vi "Teleop.vi"(10 "Match Info":T1={"Autonomous Elapsed Seconds"=0.0, "TeleOp Elapsed Seconds"=0.0, "Disabled Elapsed Seconds"=0.0, "Visited Autonomous"=FALSE, "Visited TeleOp"=FALSE, "Visited Disabled"=FALSE, "Autonomous Settings"={"Autonomous Style"=enum."Independent", "VI Refnum"=refnum}}, 11 "Call Context":T2) -> ()   [LabVIEW 2012]
doc: "This VI is called for each TeleOp packet received from the DS where the robot is not disabled. It is often used to read from the joysticks and update I/O or to update setpoints for timed control loops. It should complete and return within 20 milliseconds or it may miss DS packets."
uses:
  <vilib>/Rock Robotics/WPI/DriverStation/WPI_DriverStationDerivedRobotMode.ctl
  <vilib>/Rock Robotics/WPI/DriverStation/WPI_DriverStationMatch Info.ctl
  <vilib>/Rock Robotics/WPI/Solenoid/WPI_SolenoidValue.ctl
  Robot Global Data.vi
  <vilib>/Rock Robotics/WPI/Solenoid/WPI_SolenoidSetEnum.vi
  <vilib>/Rock Robotics/WPI/Joystick/WPI_JoystickGetSetRefNum.vi
  <vilib>/Rock Robotics/WPI/RobotDrive/WPI_RobotDriveGetSetRefNum.vi
panel:
  in  "Spin 2":dbl=0.75
  in  "Shoot 2":dbl=1.0
  in  "Spin":dbl=0.75
  in  "Shoot":dbl=1.0
  out "Numeric 1":dbl(slide) scale=0.0..100.0
  out "Boolean 2":bool
  out "Boolean 1":bool
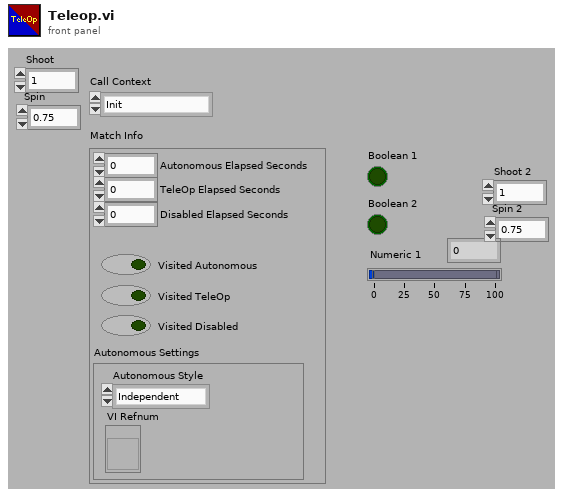
[diagram p1: front panel]
types:
  T1 = typedef "WPI_DriverStationMatch Info.ctl" = cluster{"Autonomous Elapsed Seconds":dbl, "TeleOp Elapsed Seconds":dbl, "Disabled Elapsed Seconds":dbl, "Visited Autonomous":bool, "Visited TeleOp":bool, "Visited Disabled":bool, "Autonomous Settings":cluster{"Autonomous Style":enum16{"Iterative", "Independent"}, "VI Refnum":refnum<vi>}}
  T2 = typedef "WPI_DriverStationDerivedRobotMode.ctl" = enum16{"Init", "Execute", "Stop"}
  T3 = typedef "WPI_SolenoidValue.ctl" = enum16{"Off", "On", "Forward", "Reverse"}
  T4 = typedef "WPI_RobotDriveDevRef.ctl" = cluster{"DevStatus":errorcluster, "Motors[]":T5[], "Square Inputs":bool, "Max Output":dbl, "Isochronous":bool}
  T5 = typedef "WPI_MotorControlDeviceRef.ctl" = cluster{"DeviceStatus":errorcluster, "Type":enum16{"PWM", "CAN"}, "PWM":cluster{"Digital Module":T6, "PWM Channel":T7, "DeadBand":T8}, "CAN":cluster{"Device Number":u8, "Control Mode":T9, "Semaphore":T10, "Max Vout":dbl}, "Invert":bool, "TransformRef":T11, "InvTransformRef":T11}
  T6 = typedef "FPGA_TypedefDigitalModule.ctl" = enum16{"Digital Module 1", "Digital Module 2"}
  T7 = typedef "FPGA_DIOPWMChannel.ctl" = enum8{"PWM 1", "PWM 2", "PWM 3", "PWM 4", "PWM 5", "PWM 6", "PWM 7", "PWM 8", "PWM 9", "PWM 10", "Invalid"}
  T8 = typedef "WPI_PWMDeadband.ctl" = cluster{"Name":string, "maxPositivePwm":i32, "minPositivePwm":i32, "centerPwm":i32, "maxNegativePwm":i32, "minNegativePwm":i32, "angularRange":u16}
  T9 = typedef "WPI_CANJaguar_ControlMode.ctl" = enum8{"Percent VBus", "Current", "Speed", "Position", "Voltage"}
  T10 = typedef "Semaphore RefNum" = refnum<k1>
  T11 = typedef "WPI_PWMTransform_ConPane.ctl" = refnum<vi>
  T12 = typedef "WPI_JoystickDevRef.ctl" = cluster{"Device":T13}
  T13 = typedef "WPI_JoystickDeviceEnum.ctl" = enum16{"USB 1", "USB 2", "USB 3", "USB 4", "Kinect 1", "Kinect 2"}
  T14 = typedef "WPI_JoystickButtonState.ctl" = cluster{"Button 1":bool, "Button 2":bool, "Button 3":bool, "Button 4":bool, "Button 5":bool, "Button 6":bool, "Button 7":bool, "Button 8":bool, "Button 9":bool, "Button 10":bool, "Button 11":bool, "Button 12":bool}
  T15 = cluster{"axis 1 (x)":dbl, "axis 2 (y)":dbl, "axis 3 (throttle)":dbl, "axis 4":dbl, "axis 5":dbl, "axis 6":dbl}
  T16 = typedef "WPI_SolenoidDevRef.ctl" = cluster{"DevStatus":errorcluster, "Solenoid Module":T17, "Forward Solenoid Channel":T18, "Reverse Solenoid Channel":T18}
  T17 = typedef "FPGA_TypedefSolenoidModule.ctl" = enum16{"Solenoid Module 1", "Solenoid Module 2"}
  T18 = typedef "WPI_SolenoidChannel.ctl" = enum8{"Solenoid 1", "Solenoid 2", "Solenoid 3", "Solenoid 4", "Solenoid 5", "Solenoid 6", "Solenoid 7", "Solenoid 8", "Invalid"}
  T19 = typedef "WPI_GyroDevRef.ctl" = cluster{"DevStatus":errorcluster, "Analog Module":T20, "Analog Channel":T21, "Offset":dbl, "Gain (VoltsPerDegree/Second)":dbl}
  T20 = typedef "FPGA_TypedefAnalogModule.ctl" = enum16{"Analog Module 1", "Analog Module 2"}
  T21 = typedef "FPGA_AIChannel.ctl" = enum8{"AI 1", "AI 2", "AI 3", "AI 4", "AI 5", "AI 6", "AI 7", "AI 8", "Invalid"}
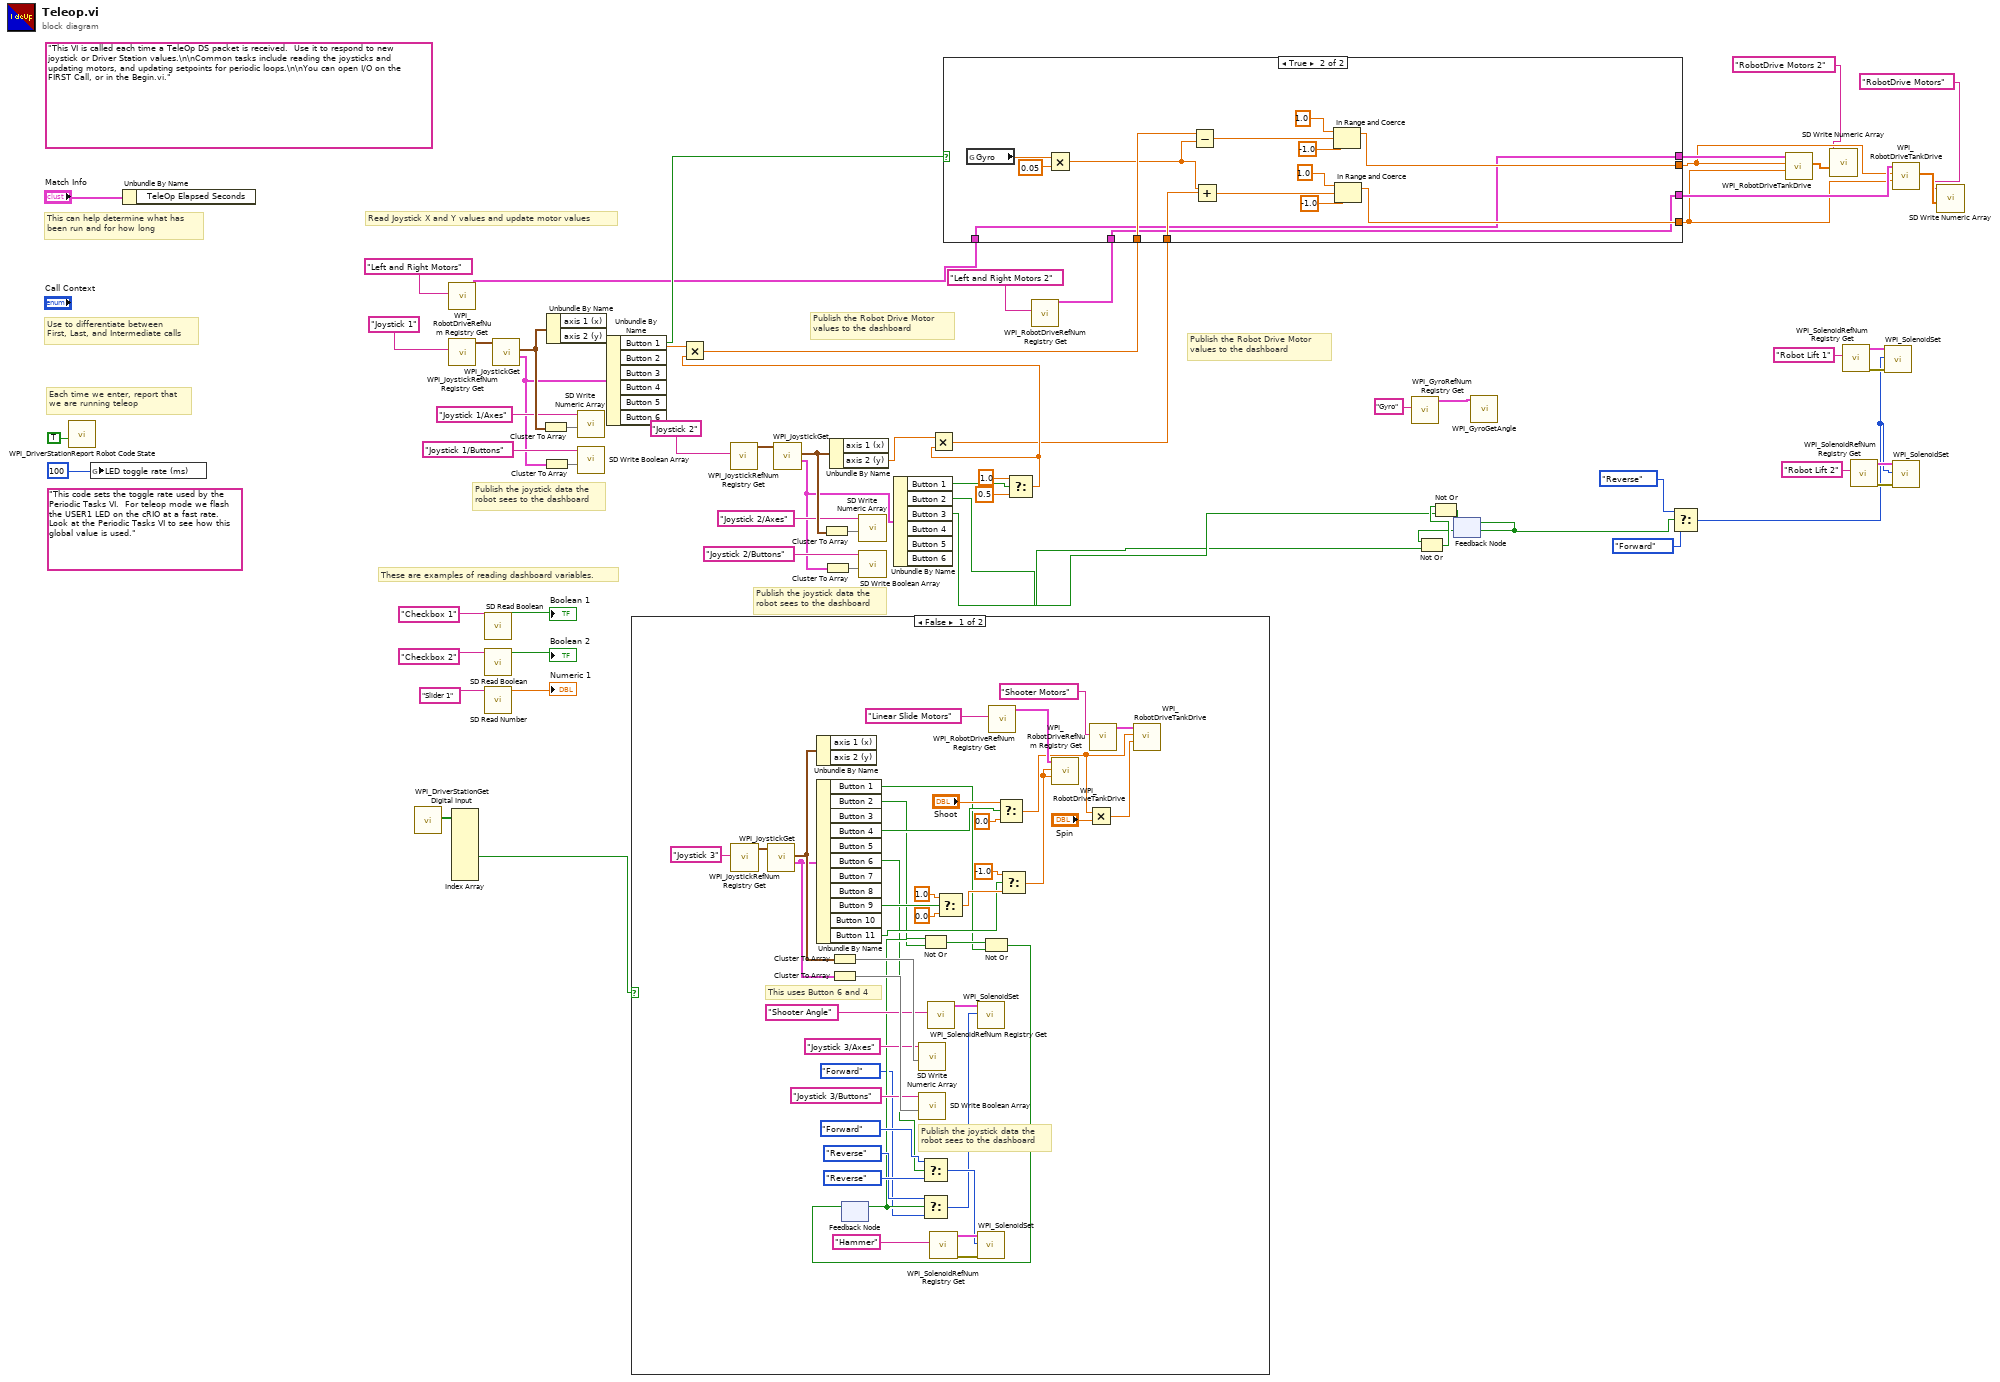
[diagram p0: block diagram]
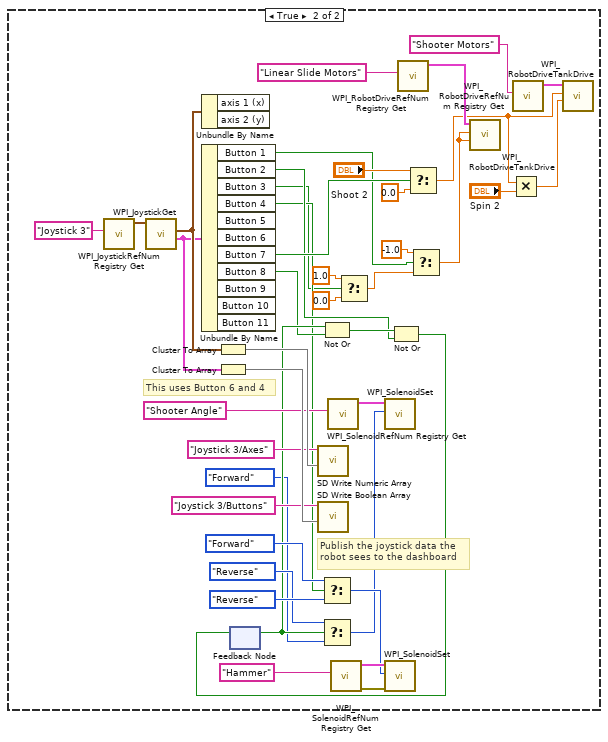
[diagram p2: hidden frame]
diagram:
  (unwired) "This code sets the toggle rate used by the Periodic Tasks VI.  For teleop mode we flash the USER1 LED on the cRIO at a fast rate.  Look at the Periodic Tasks VI to see how this global value is used."
  (unwired) "This VI is called each time a TeleOp DS packet is received.  Use it to respond to new joystick or Driver Station values.\n\nCommon tasks include reading the joysticks and updating motors, and updating setpoints for periodic loops.\n\nYou can open I/O on the FIRST Call, or in the Begin.vi."
  # "Publish the Robot Drive Motor\nvalues to the dashboard"
  # "Publish the joystick data the\nrobot sees to the dashboard"
  # "These are examples of reading dashboard variables."
  # "Publish the Robot Drive Motor\nvalues to the dashboard"
  # "Publish the joystick data the\nrobot sees to the dashboard"
  # "Each time we enter, report that\nwe are running teleop"
  # "Use to differentiate between\nFirst, Last, and Intermediate calls"
  # "This can help determine what has\nbeen run and for how long"
  # "Read Joystick X and Y values and update motor values"
  n1 = call <vilib>:"WPI_DriverStationReport Robot Code State.vi"("TeleOp"=TRUE ("Autonomous")) -> ()  [unwired: 10 in, 1 out]
  n2 = global write "Robot Global Data.vi" "LED toggle rate (ms)"(u32 100 ("LED ms toggle rate")) -> ()
  n3 = Unbundle By Name("Match Info") -> ()  [unwired: 1 out]
  n4 = call <vilib>:"WPI_DriverStationGet Digital Input.vi"() -> ("Driver Station Digital Input (1-8)"=w2:bool[])  [unwired: 11 out]
  n5 = call <vilib>:"WPI_RobotDriveRefNum Registry Get.vi"("refnum name"="Left and Right Motors") -> ("RobotDriveDevRef"=w17:T4)  [unwired: 1 in, 9 out]
  n6 = call <vilib>:"WPI_JoystickRefNum Registry Get.vi"("refnum name"="Joystick 1") -> ("JoystickDevRef"=w61:T12)  [unwired: 1 in, 9 out]
  n7 = Index Array(array=w2) -> (element #5=w1:bool)  [unwired: 8 in, 7 out]
  n8 = call <vilib>:"SD Read Boolean.vi"("Name"="Checkbox 1" ("refnum name")) -> ("Boolean"=→"Boolean 1":bool)  [unwired: 8 in, 2 out]
  n9 = call <vilib>:"SD Read Boolean.vi"("Name"="Checkbox 2" ("refnum name")) -> ("Boolean"=→"Boolean 2":bool)  [unwired: 8 in, 2 out]
  n10 = call <vilib>:"SD Read Number.vi"("Name"="Slider 1" ("refnum name")) -> ("Numeric"=→"Numeric 1":dbl)  [unwired: 8 in, 2 out]
  n11 = call <vilib>:"WPI_JoystickGet.vi"("JoystickDevRef"=w61) -> ("Buttons"=w19:T14, "Axes"=w56:T15)  [unwired: 1 in, 4 out]
  n12 = Cluster To Array(cluster=w56) -> (array=w55:dbl[])
  n13 = Cluster To Array(cluster=w19) -> (array=w58:bool[])
  n14 = Unbundle By Name(w56) -> ("axis 2 (y)"=w35:dbl)  [unwired: 1 out]
  n15 = call <vilib>:"SD Write Numeric Array.vi"("Numeric Array"=w55, "Name"="Joystick 1/Axes") -> ()  [unwired: 8 in, 2 out]
  n16 = call <vilib>:"SD Write Boolean Array.vi"("Boolean Array"=w58, "Name"="Joystick 1/Buttons") -> ()  [unwired: 8 in, 2 out]
  n17 = Unbundle By Name(w19) -> ("Button 1"=w18:bool)  [unwired: 5 out]
  n18 = case shown="False" w1 {
    frame False {
      # "This uses Button 6 and 4"
      # "Publish the joystick data the\nrobot sees to the dashboard"
      n19 = call <vilib>:"WPI_JoystickRefNum Registry Get.vi"("refnum name"="Joystick 3") -> ("JoystickDevRef"=w104:T12)  [unwired: 1 in, 9 out]
      n20 = call <vilib>:"WPI_JoystickGet.vi"("JoystickDevRef"=w104) -> ("Buttons"=w98:T14, "Axes"=w101:T15)  [unwired: 1 in, 4 out]
      n21 = Unbundle By Name(w101) -> ()  [unwired: 2 out]
      n22 = Unbundle By Name(w98) -> ("Button 1"=w65:bool, "Button 2"=w67:bool, "Button 4"=w68:bool, "Button 6"=w66:bool, "Button 9"=w69:bool, "Button 11"=w93:bool)  [unwired: 5 out]
      n23 = Cluster To Array(cluster=w101) -> (array=w100:dbl[])
      n24 = Cluster To Array(cluster=w98) -> (array=w103:bool[])
      n25 = feedback #1() -> (w71:bool)  [unwired: 1 in]
      n26 = call <vilib>:"SD Write Numeric Array.vi"("Numeric Array"=w100, "Name"="Joystick 3/Axes") -> ()  [unwired: 8 in, 2 out]
      n27 = call <vilib>:"SD Write Boolean Array.vi"("Boolean Array"=w103, "Name"="Joystick 3/Buttons") -> ()  [unwired: 8 in, 2 out]
      n28 = Not Or(1:w67, 2:w71) -> (0:w73:bool)
      n29 = Select(t=WPI_SolenoidValue."Forward" ("Value"), s=w66, f=WPI_SolenoidValue."Reverse" ("Value")) -> (s? t:f=w80:T3)
      n30 = Select(t=WPI_SolenoidValue."Reverse" ("Value"), s=w71, f=WPI_SolenoidValue."Forward" ("Value")) -> (s? t:f=w75:T3)
      n31 = call <vilib>:"WPI_SolenoidRefNum Registry Get.vi"("refnum name"="Shooter Angle") -> ("SolenoidDevRef"=w76:T16)  [unwired: 9 in, 1 out]
      n32 = call <vilib>:"WPI_SolenoidRefNum Registry Get.vi"("refnum name"="Hammer") -> ("error out"=w83:errorcluster, "SolenoidDevRef"=w82:T16)  [unwired: 9 in]
      n33 = Select(t=1.0, s=w69, f=0.0) -> (s? t:f=w94:dbl)
      n34 = call-poly <vilib>:"WPI_SolenoidSet.vi"("Value"=w75, "SolenoidDevRef"=w76) -> ()  [unwired: 8 in, 2 out]
      n35 = call-poly <vilib>:"WPI_SolenoidSet.vi"("error in (no error)"=w83, "Value"=w80, "SolenoidDevRef"=w82) -> ()  [unwired: 7 in, 2 out]
      n36 = Not Or(1:w65, 2:w73) -> (0:w72:bool)
      n37 = feedback-in #1(w72) -> ()
      n38 = call <vilib>:"WPI_RobotDriveRefNum Registry Get.vi"("refnum name"="Linear Slide Motors") -> ("RobotDriveDevRef"=w91:T4)  [unwired: 9 in, 1 out]
      n39 = Select(t="Shoot", s=w68, f=0.0) -> (s? t:f=w85:dbl)
      n40 = Select(t=-1.0, s=w93, f=w94) -> (s? t:f=w92:dbl)
      n41 = call <vilib>:"WPI_RobotDriveTankDrive.vi"("Right axis value"=w92, "Left axis value"=w92, "RobotDriveDevRef"=w91) -> ()  [unwired: 6 in, 3 out]
      n42 = Multiply(x=w85, y="Spin") -> (x*y=w84:dbl)
      n43 = call <vilib>:"WPI_RobotDriveRefNum Registry Get.vi"("refnum name"="Shooter Motors") -> ("RobotDriveDevRef"=w89:T4)  [unwired: 9 in, 1 out]
      n44 = call <vilib>:"WPI_RobotDriveTankDrive.vi"("Right axis value"=w84, "Left axis value"=w85, "RobotDriveDevRef"=w89) -> ()  [unwired: 6 in, 3 out]
    }
    frame True {
      # "This uses Button 6 and 4"
      # "Publish the joystick data the\nrobot sees to the dashboard"
      n45 = call <vilib>:"WPI_JoystickRefNum Registry Get.vi"("refnum name"="Joystick 3") -> ("JoystickDevRef"=w146:T12)  [unwired: 1 in, 9 out]
      n46 = call <vilib>:"WPI_JoystickGet.vi"("JoystickDevRef"=w146) -> ("Buttons"=w140:T14, "Axes"=w143:T15)  [unwired: 1 in, 4 out]
      n47 = Unbundle By Name(w143) -> ()  [unwired: 2 out]
      n48 = Unbundle By Name(w140) -> ("Button 1"=w107:bool, "Button 2"=w110:bool, "Button 3"=w108:bool, "Button 4"=w109:bool, "Button 7"=w112:bool, "Button 8"=w111:bool)  [unwired: 5 out]
      n49 = Cluster To Array(cluster=w143) -> (array=w142:dbl[])
      n50 = Cluster To Array(cluster=w140) -> (array=w145:bool[])
      n51 = feedback #2() -> (w114:bool)  [unwired: 1 in]
      n52 = call <vilib>:"SD Write Numeric Array.vi"("Numeric Array"=w142, "Name"="Joystick 3/Axes") -> ()  [unwired: 8 in, 2 out]
      n53 = call <vilib>:"SD Write Boolean Array.vi"("Boolean Array"=w145, "Name"="Joystick 3/Buttons") -> ()  [unwired: 8 in, 2 out]
      n54 = Not Or(1:w111, 2:w114) -> (0:w116:bool)
      n55 = Select(t=WPI_SolenoidValue."Forward" ("Value"), s=w109, f=WPI_SolenoidValue."Reverse" ("Value")) -> (s? t:f=w123:T3)
      n56 = Select(t=WPI_SolenoidValue."Reverse" ("Value"), s=w114, f=WPI_SolenoidValue."Forward" ("Value")) -> (s? t:f=w118:T3)
      n57 = call <vilib>:"WPI_SolenoidRefNum Registry Get.vi"("refnum name"="Shooter Angle") -> ("SolenoidDevRef"=w119:T16)  [unwired: 9 in, 1 out]
      n58 = call <vilib>:"WPI_SolenoidRefNum Registry Get.vi"("refnum name"="Hammer") -> ("error out"=w126:errorcluster, "SolenoidDevRef"=w125:T16)  [unwired: 9 in]
      n59 = Select(t=1.0, s=w108, f=0.0) -> (s? t:f=w136:dbl)
      n60 = call-poly <vilib>:"WPI_SolenoidSet.vi"("Value"=w118, "SolenoidDevRef"=w119) -> ()  [unwired: 8 in, 2 out]
      n61 = call-poly <vilib>:"WPI_SolenoidSet.vi"("error in (no error)"=w126, "Value"=w123, "SolenoidDevRef"=w125) -> ()  [unwired: 7 in, 2 out]
      n62 = Not Or(1:w110, 2:w116) -> (0:w115:bool)
      n63 = feedback-in #2(w115) -> ()
      n64 = call <vilib>:"WPI_RobotDriveRefNum Registry Get.vi"("refnum name"="Linear Slide Motors") -> ("RobotDriveDevRef"=w134:T4)  [unwired: 9 in, 1 out]
      n65 = Select(t="Shoot 2", s=w112, f=0.0) -> (s? t:f=w128:dbl)
      n66 = Select(t=-1.0, s=w107, f=w136) -> (s? t:f=w135:dbl)
      n67 = call <vilib>:"WPI_RobotDriveTankDrive.vi"("Right axis value"=w135, "Left axis value"=w135, "RobotDriveDevRef"=w134) -> ()  [unwired: 6 in, 3 out]
      n68 = Multiply(x=w128, y="Spin 2") -> (x*y=w127:dbl)
      n69 = call <vilib>:"WPI_RobotDriveRefNum Registry Get.vi"("refnum name"="Shooter Motors") -> ("RobotDriveDevRef"=w132:T4)  [unwired: 9 in, 1 out]
      n70 = call <vilib>:"WPI_RobotDriveTankDrive.vi"("Right axis value"=w127, "Left axis value"=w128, "RobotDriveDevRef"=w132) -> ()  [unwired: 6 in, 3 out]
    }
  }
  n71 = call <vilib>:"WPI_JoystickRefNum Registry Get.vi"("refnum name"="Joystick 2") -> ("JoystickDevRef"=w46:T12)  [unwired: 1 in, 9 out]
  n72 = call <vilib>:"WPI_JoystickGet.vi"("JoystickDevRef"=w46) -> ("Buttons"=w39:T14, "Axes"=w43:T15)  [unwired: 1 in, 4 out]
  n73 = Cluster To Array(cluster=w43) -> (array=w42:dbl[])
  n74 = Cluster To Array(cluster=w39) -> (array=w45:bool[])
  n75 = Unbundle By Name(w43) -> ("axis 2 (y)"=w34:dbl)  [unwired: 1 out]
  n76 = call <vilib>:"SD Write Numeric Array.vi"("Numeric Array"=w42, "Name"="Joystick 2/Axes") -> ()  [unwired: 8 in, 2 out]
  n77 = call <vilib>:"SD Write Boolean Array.vi"("Boolean Array"=w45, "Name"="Joystick 2/Buttons") -> ()  [unwired: 8 in, 2 out]
  n78 = Unbundle By Name(w39) -> ("Button 1"=w38:bool, "Button 2"=w4:bool, "Button 3"=w5:bool)  [unwired: 3 out]
  n79 = Select(t=1.0, s=w38, f=0.5) -> (s? t:f=w33:dbl)
  n80 = Multiply(x=w35, y=w33) -> (x*y=w15:dbl)
  n81 = Multiply(x=w34, y=w33) -> (x*y=w6:dbl)
  n82 = call <vilib>:"WPI_RobotDriveRefNum Registry Get.vi"("refnum name"="Left and Right Motors 2") -> ("RobotDriveDevRef"=w16:T4)  [unwired: 1 in, 9 out]
  n83 = case shown="True" w18 {
    tunnel: w17 -> [w152 w153]
    tunnel: w16 -> [w151 w154]
    tunnel: w15 -> [w150 w162]
    tunnel: [w149 w155] -> w7
    tunnel: [w152 w153] -> w12
    tunnel: [w151 w154] -> w11
    tunnel: [w150 w156] -> w10
    tunnel: w6 -> [w149 w163]
    frame False {
    }
    frame True {
      n84 = global read "Robot Global Data.vi" "Gyro"() -> (w167:dbl)
      n85 = Multiply(x=w167, y=0.05) -> (x*y=w161:dbl)
      n86 = Subtract(x=w162, y=w161) -> (x-y=w160:dbl)
      n87 = Add(x=w161, y=w163) -> (x+y=w157:dbl)
      n88 = In Range and Coerce(upper limit=1.0, x=w160, lower limit=-1.0) -> (coerced(x)=w156:dbl)  [unwired: 1 out]
      n89 = In Range and Coerce(upper limit=1.0, x=w157, lower limit=-1.0) -> (coerced(x)=w155:dbl)  [unwired: 1 out]
    }
  }
  n90 = call <vilib>:"WPI_GyroRefNum Registry Get.vi"("refnum name"="Gyro") -> ("GyroDevRef"=w21:T19)  [unwired: 9 in, 1 out]
  n91 = feedback #3() -> (w22:bool)  [unwired: 1 in]
  n92 = Not Or(1:w4, 2:w22) -> (0:w24:bool)
  n93 = Not Or(1:w5, 2:w24) -> (0:w23:bool)
  n94 = feedback-in #3(w23) -> ()
  n95 = call <vilib>:"WPI_GyroGetAngle.vi"("GyroDevRef"=w21) -> ()  [unwired: 7 in, 4 out]
  n96 = Select(t=WPI_SolenoidValue."Reverse" ("Value"), s=w22, f=WPI_SolenoidValue."Forward" ("Value")) -> (s? t:f=w25:T3)
  n97 = call <vilib>:"WPI_RobotDriveTankDrive.vi"("Right axis value"=w7, "Left axis value"=w10, "RobotDriveDevRef"=w12) -> ("Motor Values"=w13:dbl[])  [unwired: 6 in, 2 out]
  n98 = call <vilib>:"SD Write Numeric Array.vi"("Numeric Array"=w13, "Name"="RobotDrive Motors 2") -> ()  [unwired: 8 in, 2 out]
  n99 = call <vilib>:"WPI_SolenoidRefNum Registry Get.vi"("refnum name"="Robot Lift 1") -> ("error out"=w32:errorcluster, "SolenoidDevRef"=w31:T16)  [unwired: 9 in]
  n100 = call <vilib>:"WPI_SolenoidRefNum Registry Get.vi"("refnum name"="Robot Lift 2") -> ("error out"=w29:errorcluster, "SolenoidDevRef"=w28:T16)  [unwired: 9 in]
  n101 = call-poly <vilib>:"WPI_SolenoidSet.vi"("error in (no error)"=w32, "Value"=w25, "SolenoidDevRef"=w31) -> ()  [unwired: 7 in, 2 out]
  n102 = call <vilib>:"WPI_RobotDriveTankDrive.vi"("Right axis value"=w7, "Left axis value"=w10, "RobotDriveDevRef"=w11) -> ("Motor Values"=w14:dbl[])  [unwired: 6 in, 2 out]
  n103 = call-poly <vilib>:"WPI_SolenoidSet.vi"("error in (no error)"=w29, "Value"=w25, "SolenoidDevRef"=w28) -> ()  [unwired: 7 in, 2 out]
  n104 = call <vilib>:"SD Write Numeric Array.vi"("Numeric Array"=w14, "Name"="RobotDrive Motors") -> ()  [unwired: 8 in, 2 out]
